vi "Constructor.vi"(5 "TimeZoneInfoId":string, 6 "OperationStatus":T1=enum."NOT_COMPLETED", 7 "OperationRunStartTime":timestamp, 8 "error in":errorcluster, 9 "OperationName":string, 10 "ProcessFullName":string, 11 "Name":string) -> (0 "error out":errorcluster, 3 "OperationRun out":refnum<class "OperationRun.lvclass">)   [LabVIEW 2021, in "ProligentXMLGenerator.lvlib" / "OperationRun.lvclass"]
uses:
  OperationRun.lvclass
  OperationRun.lvclass/OperationRun.ctl
  Base/DateTime/DateTime.lvclass
  Base/ProcessFullName/ProcessFullName.lvclass
  Base/NonEmptyString_65/NonEmptyString_65.lvclass
  Base/ExecutionStatus/ExecutionStatus.lvclass
  Data.ctl
  SequenceRun/SequenceRun/SequenceRun.lvclass
  Base/NonEmptyString_255/NonEmptyString_255.lvclass
  Base/Guid/Guid.lvclass
  Base/FullName/FullName.lvclass
  Base/NonEmptyString_64/NonEmptyString_64.lvclass
  Model/CustomData/CustomData.lvclass
  SequenceRun/SequenceRunReference/SequenceRunReference.lvclass
  Failure/FailureReference/FailureReference.lvclass
  Model/Document/Document.lvclass
  Model/Characteristic/Characteristic.lvclass
  Base/ExecutionStatus/Value.ctl
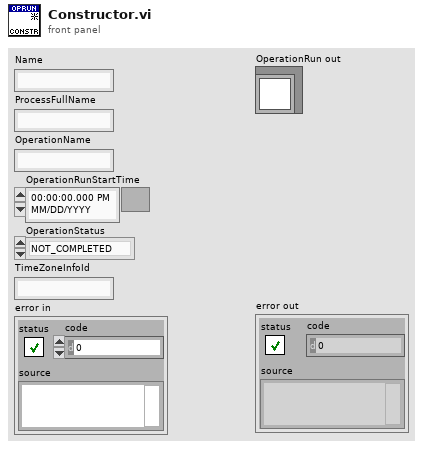
[diagram p1: front panel]
types:
  T1 = typedef "ProligentXMLGenerator.lvlib/ExecutionStatus.lvclass/Value.ctl" = enum16{"PASS", "FAIL", "NOT_COMPLETED", "ABORTED"}
  T2 = typedef "ProligentXMLGenerator.lvlib/OperationRun.lvclass/Data.ctl" = cluster{"Name":string, "Characteristics":refnum<class "Characteristic.lvclass">[], "Documents":refnum<class "Document.lvclass">[], "SequenceRuns":refnum<class "SequenceRun.lvclass">[], "FailureReferences":refnum<class "FailureReference.lvclass">[], "SequenceRunReferences":refnum<class "SequenceRunReference.lvclass">[], "CustomData":refnum<class "CustomData.lvclass">, "OperationRunId":refnum<class "Guid.lvclass">, "ProcessFullName":refnum<class "ProcessFullName.lvclass">, "ProcessVersion":refnum<class "NonEmptyString_64.lvclass">, "OperationName":refnum<class "NonEmptyString_65.lvclass">, "StationFullName":refnum<class "FullName.lvclass">, "User":refnum<class "NonEmptyString_255.lvclass">, "CallingOperationRunId":refnum<class "Guid.lvclass">, "OperationStatus":refnum<class "ExecutionStatus.lvclass">, "OperationRunStartTime":refnum<class "DateTime.lvclass">, "OperationRunEndTime":refnum<class "DateTime.lvclass">, "TimeZoneInfoId":string}
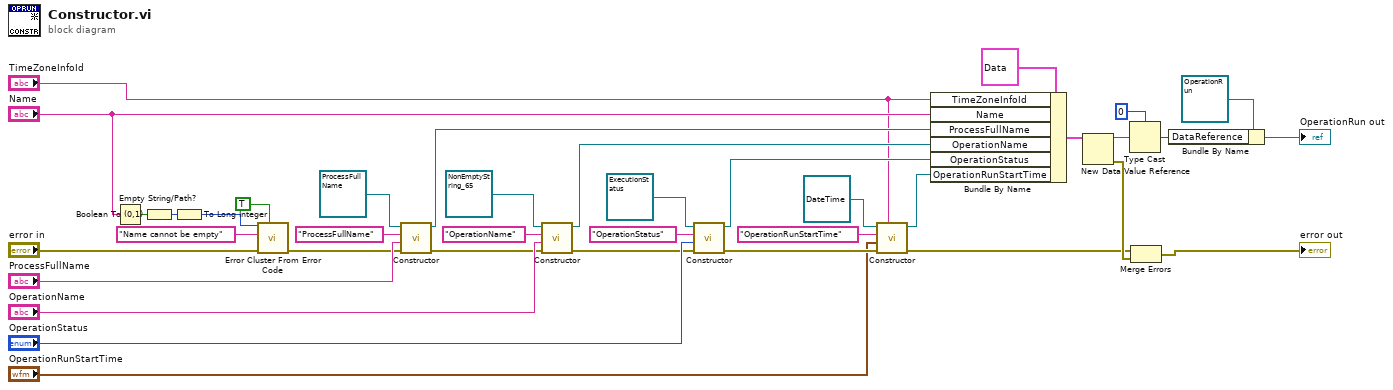
[diagram p0: block diagram]
diagram:
  n1 = Empty String/Path?(string/path="Name") -> (empty?=w22:bool)
  n2 = Boolean To (0,1)(Boolean=w22) -> (0, 1=w21:i16)
  n3 = To Long Integer(number=w21) -> (32bit integer=w20:i32)
  n4 = call <vilib>:"Error Cluster From Error Code.vi"("show call chain? (False)"=TRUE, "error in (no error)"="error in", "error message (\"\")"="Name cannot be empty" ("error message (\"\")"), "error code (0)"=w20) -> ("error out"=w16:errorcluster)  [unwired: 5 in]
  n5 = call-dynamic "Constructor.vi"("error in"=w16, "Value"="ProcessFullName", "Name"="ProcessFullName", "String in"=refnum<class "ProcessFullName.lvclass"> refnum ("ProligentResultProcessor:ProcessFullName")) -> ("error out"=w11:errorcluster, "String out"=w17:refnum<class "ProcessFullName.lvclass">)  [unwired: 6 in]
  n6 = call-dynamic "Constructor.vi"("error in"=w11, "Value"="OperationName", "Name"="OperationName", "String in"=refnum<class "NonEmptyString_65.lvclass"> refnum ("ProligentResultProcessor:NonEmptyString_65")) -> ("error out"=w8:errorcluster, "String out"=w10:refnum<class "NonEmptyString_65.lvclass">)  [unwired: 6 in]
  n7 = call-dynamic "Constructor.vi"("error in"=w8, "Value"="OperationStatus", "Name"="OperationStatus", "ExecutionStatus in"=refnum<class "ExecutionStatus.lvclass"> refnum ("ProligentResultProcessor:ExecutionStatus")) -> ("error out"=w7:errorcluster, "ExecutionStatus out"=w4:refnum<class "ExecutionStatus.lvclass">)  [unwired: 6 in]
  n8 = call-dynamic "Constructor.vi"("TimeZoneInfoId"="TimeZoneInfoId", "error in"=w7, "Value"="OperationRunStartTime", "Name"="OperationRunStartTime", "DateTime in"=refnum<class "DateTime.lvclass"> refnum) -> ("error out"=w15:errorcluster, "DateTime out"=w24:refnum<class "DateTime.lvclass">)  [unwired: 5 in]
  n9 = Bundle By Name(cluster=T2 {"Name"="", "Characteristics"=[], "Documents"=[], "SequenceRuns"=[], "FailureReferences"=[], "SequenceRunReferences"=[], "CustomData"=refnum, "OperationRunId"=refnum, "ProcessFullName"=refnum, "ProcessVersion"=refnum, "OperationName"=refnum, "StationFullName"=refnum, "User"=refnum, "CallingOperationRunId"=refnum, "OperationStatus"=refnum, "OperationRunStartTime"=refnum, "OperationRunEndTime"=refnum, "TimeZoneInfoId"=""} ("Data"), "TimeZoneInfoId"="TimeZoneInfoId", "Name"="Name", "ProcessFullName"=w17, "OperationName"=w10, "OperationStatus"=w4, "OperationRunStartTime"=w24) -> (w29:T2)
  n10 = New Data Value Reference(data value=w29) -> (data value reference=w28:refnum<data-value>, error out=w25:errorcluster)  [unwired: 1 in]
  n11 = Type Cast(type=u64 0, x=w28) -> (*(type *) &x=w26:u64)
  n12 = Merge Errors(w15, w25) -> (→"error out":errorcluster)
  n13 = Bundle By Name(cluster=refnum<class "OperationRun.lvclass"> refnum ("ProligentResultProcessor:OperationRun"), "DataReference"=w26) -> (→"OperationRun out":refnum<class "OperationRun.lvclass">)
